vi "Execute.vi"(8 "error in (no error)":errorcluster, 9 "Workspace":T1, 10 "Control In":T2={"I-O.lvclass"=refnum, "Motion.lvclass"=refnum, "Dispenser.lvclass"=refnum}, 11 "Secure Syringe in":refnum<class "SecureRelease Syringe.lvclass">) -> (0 "error out":errorcluster, 2 "Control Out":T2, 3 "Secure Syringe out":refnum<class "SecureRelease Syringe.lvclass">)   [LabVIEW 2016, in "SecureRelease Syringe.lvclass"]
uses:
  SecureRelease Syringe.lvclass
  Controller/Controllers.ctl
  Controller/I-O/I-O.lvclass
  Controller/Motion/A3200/A3200.lvclass
  Controller/Dispenser/Dispenser.lvclass
  Controller/Motion/Motion.lvclass
  Workspace/Workspace.ctl
  SecureRelease Syringe.lvclass/SecureRelease Syringe.ctl
  Dispense/Dispense.lvclass
  Controller/Controller.lvclass
  Workspace/Fixture.lvclass
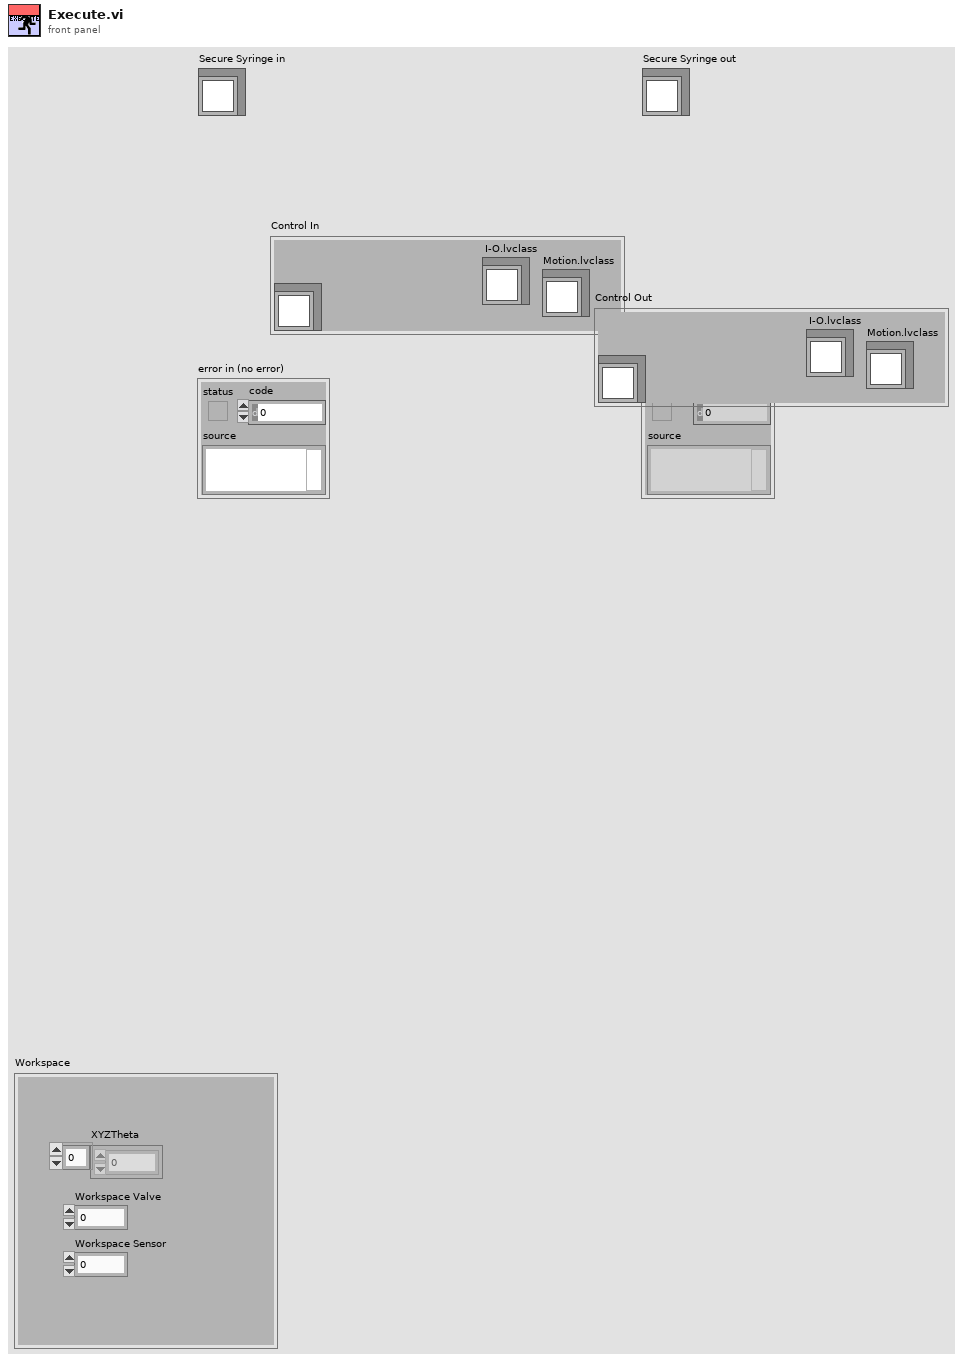
[diagram p1: front panel]
types:
  T1 = typedef "Fixture.lvclass/Workspace.ctl" = cluster{"XYZTheta":dbl[], "Workspace Valve":i32, "Workspace Sensor":i32}
  T2 = typedef "Controller.lvclass/Controllers.ctl" = cluster{"I-O.lvclass":refnum<class "I-O.lvclass">, "Motion.lvclass":refnum<class "Motion.lvclass">, "Dispenser.lvclass":refnum<class "Dispenser.lvclass">}
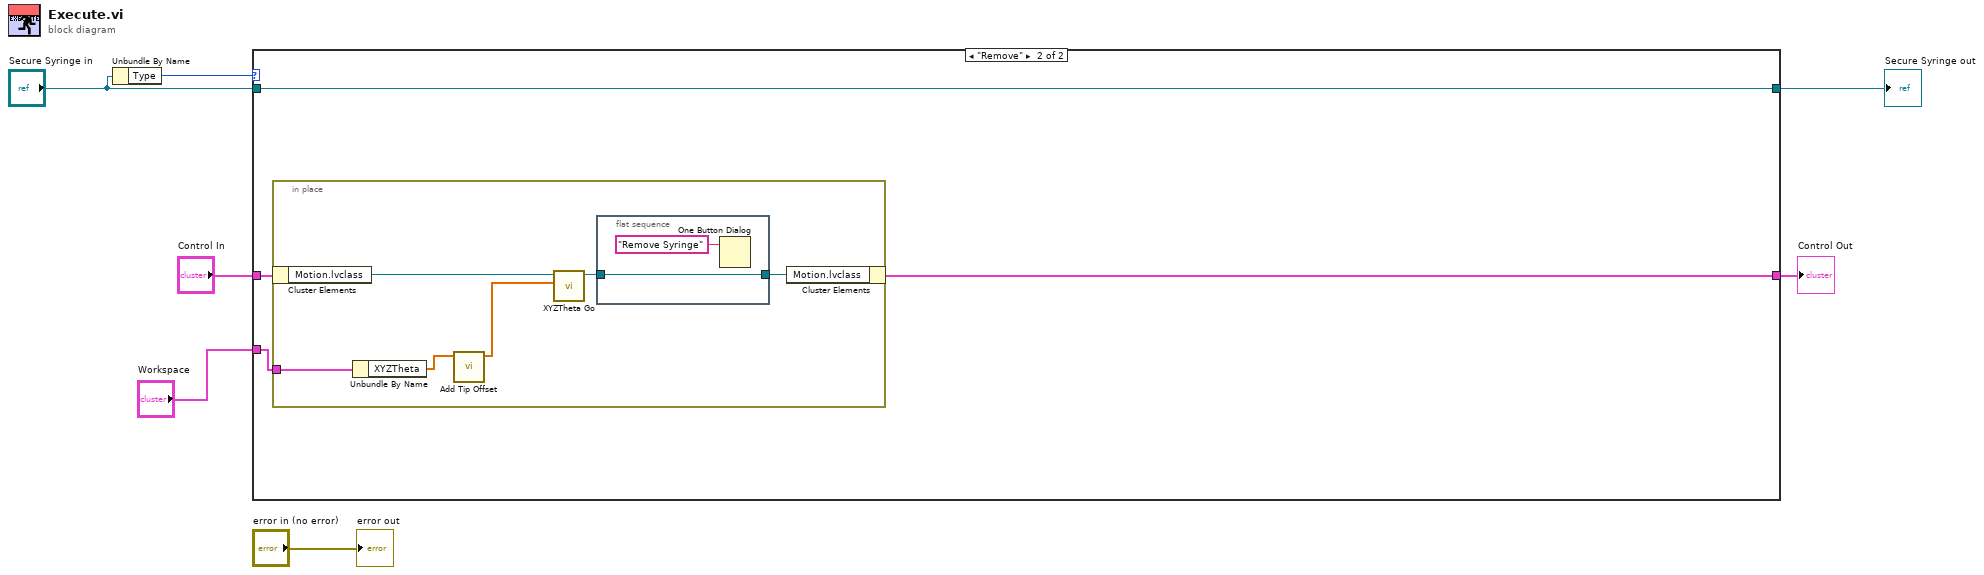
[diagram p0: block diagram]
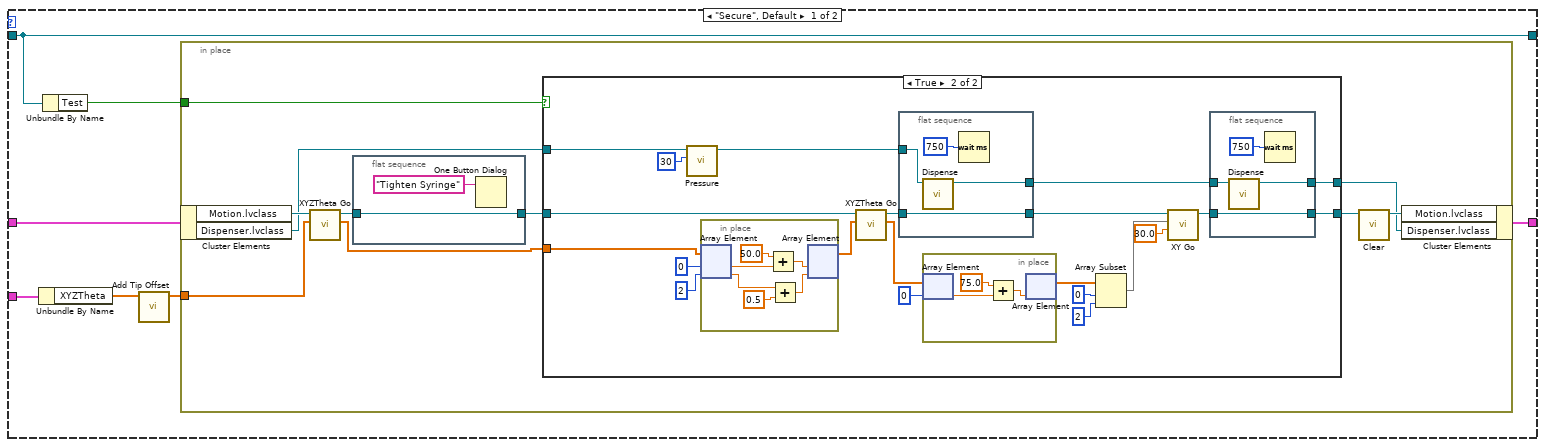
[diagram p2: hidden frame]
diagram:
  n1 = Unbundle By Name("Secure Syringe in") -> ("Type"=w1:enum16{"Secure", "Remove"})
  n2 = case shown="\"Remove\"" w1 {
    tunnel: "Workspace" -> [w14 w67]
    tunnel: "Secure Syringe in" -> [w10 w68]
    tunnel: [w10 w68] -> w5
    tunnel: "Control In" -> [w13 w69]
    tunnel: [w12 w70] -> w3
    frame "Secure", Default {
      n3 = Unbundle By Name(w14) -> ("XYZTheta"=w9:dbl[])
      n4 = Unbundle By Name(w10) -> ("Test"=w11:bool)
      n5 = call "Add Tip Offset.vi"("XYZTheta"=w9) -> ("XYZTheta"=w8:dbl[])  [unwired: 10 in]
      n6 = in-place {
        in-place-border: w8 -> [w23]
        in-place-border: w11 -> [w17]
        n7 = in-place-cluster #1(w13) -> ("Motion.lvclass"=w24:refnum<class "Motion.lvclass">, "Dispenser.lvclass"=w16:refnum<class "Dispenser.lvclass">)
        n8 = call "XYZTheta Go.vi"("XYZTheta In"=w23, "Motion in"=w24) -> ("XYZTheta Out"=w18:dbl[], "Motion out"=w22:refnum<class "Motion.lvclass">)  [unwired: 7 in, 1 out]
        n9 = flat-sequence {
          tunnel: [w65] -> w20
          tunnel: w22 -> [w65]
          frame #0 {
            n10 = One Button Dialog(message="Tighten Syringe") -> ()  [unwired: 1 in, 1 out]
          }
        }
        n11 = case shown="True" w17 {
          tunnel: w20 -> [w26 w47]
          tunnel: [w26 w33] -> w19
          tunnel: w18 -> [_ w46]
          tunnel: w16 -> [w25 w39]
          tunnel: [w25 w31] -> w15
          frame False {
          }
          frame True {
            n12 = call-dynamic "Pressure.vi"("Pressure"=i16 30, "Dispenser in"=w39) -> ("Dispenser out"=w35:refnum<class "Dispenser.lvclass">)  [unwired: 8 in, 1 out]
            n13 = in-place {
              n14 = in-place-array #2(w46, 0, 2) -> (w64:dbl, w62:dbl)
              n15 = Add(x=50.0, y=w64) -> (x+y=w59:dbl)
              n16 = Add(x=w62, y=0.5) -> (x+y=w60:dbl)
              n17 = in-place-array #2(w59, w60) -> (w43:dbl[])  [unwired: 2 out]
            }
            n18 = call "XYZTheta Go.vi"("XYZTheta In"=w43, "Motion in"=w47) -> ("XYZTheta Out"=w42:dbl[], "Motion out"=w36:refnum<class "Motion.lvclass">)  [unwired: 7 in, 1 out]
            n19 = flat-sequence {
              tunnel: [w55] -> w37
              tunnel: w36 -> [w55]
              tunnel: w35 -> [w54]
              tunnel: [w52] -> w32
              frame #0 {
                n20 = call-dynamic "Dispense.vi"("Dispenser in"=w54) -> ("Dispenser out"=w52:refnum<class "Dispenser.lvclass">)  [unwired: 9 in, 1 out]
                n21 = Wait (ms)(milliseconds to wait=u32 750) -> ()  [unwired: 1 out]
              }
            }
            n22 = in-place {
              n23 = in-place-array #3(w42, 0) -> (w58:dbl)
              n24 = Add(x=75.0, y=w58) -> (x+y=w56:dbl)
              n25 = in-place-array #3(w56) -> (w30:dbl[])  [unwired: 1 out]
            }
            n26 = Array Subset(array=w30, index=0, length=2) -> (w27:dbl[])
            n27 = call-dynamic "XY Go.vi"("Speed"=30.0, "XY"=w27, "Motion in"=w37) -> ("Motion out"=w34:refnum<class "Motion.lvclass">)  [unwired: 7 in, 1 out]
            n28 = flat-sequence {
              tunnel: [w51] -> w33
              tunnel: w34 -> [w51]
              tunnel: w32 -> [w50]
              tunnel: [w48] -> w31
              frame #0 {
                n29 = call-dynamic "Dispense.vi"("Dispenser in"=w50) -> ("Dispenser out"=w48:refnum<class "Dispenser.lvclass">)  [unwired: 9 in, 1 out]
                n30 = Wait (ms)(milliseconds to wait=u32 750) -> ()  [unwired: 1 out]
              }
            }
          }
        }
        n31 = call "Clear.vi"("Motion in"=w19) -> ("Motion out"=w21:refnum<class "Motion.lvclass">)  [unwired: 9 in, 1 out]
        n32 = in-place-cluster #1("Motion.lvclass"=w21, "Dispenser.lvclass"=w15) -> (w12:T2)
      }
    }
    frame "Remove" {
      n33 = in-place {
        in-place-border: w67 -> [w73]
        n34 = in-place-cluster #4(w69) -> ("Motion.lvclass"=w76:refnum<class "Motion.lvclass">)
        n35 = Unbundle By Name(w73) -> ("XYZTheta"=w72:dbl[])
        n36 = call "Add Tip Offset.vi"("XYZTheta"=w72) -> ("XYZTheta"=w71:dbl[])  [unwired: 10 in]
        n37 = call "XYZTheta Go.vi"("XYZTheta In"=w71, "Motion in"=w76) -> ("Motion out"=w75:refnum<class "Motion.lvclass">)  [unwired: 7 in, 2 out]
        n38 = flat-sequence {
          tunnel: w75 -> [w78]
          tunnel: [w78] -> w74
          frame #0 {
            n39 = One Button Dialog(message="Remove Syringe") -> ()  [unwired: 1 in, 1 out]
          }
        }
        n40 = in-place-cluster #4("Motion.lvclass"=w74) -> (w70:T2)
      }
    }
  }
  "Secure Syringe out" <- w5
  "Control Out" <- w3
  "error out" <- "error in (no error)"
